vi "Average_data.vi"(7 "Data for averaging":dbl[][](array[numeric]), 8 "error in (no error)":errorcluster, 9 "Number to average":i32, 10 "New data":dbl[](array[numeric]), 11 "Gage digitizer actor in":refnum<class "Gage digitizer actor.lvclass">) -> (0 "error out":errorcluster, 2 "Aveage data":dbl[](array[numeric]), 3 "Gage digitizer actor out":refnum<class "Gage digitizer actor.lvclass">)   [LabVIEW 2015, in "Gage digitizer actor.lvclass"]
uses:
  Gage digitizer actor.lvclass
  <vilib>/Analysis/baseanly.llb/Mean (DBL).vi
  <vilib>/Analysis/NI_AALBase.lvlib
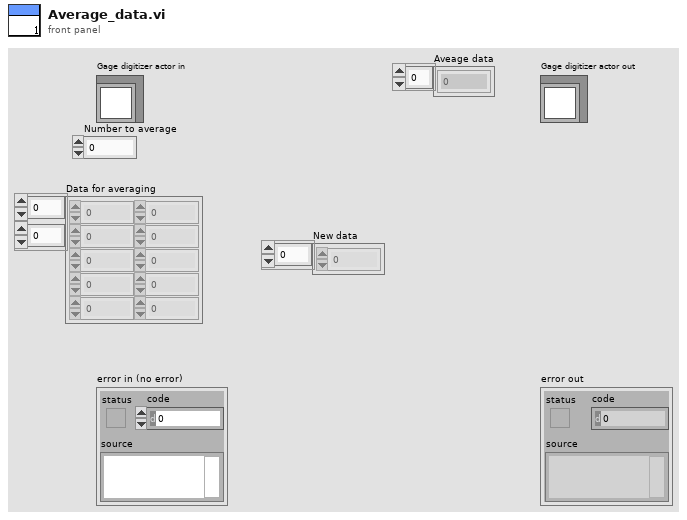
[diagram p1: front panel]
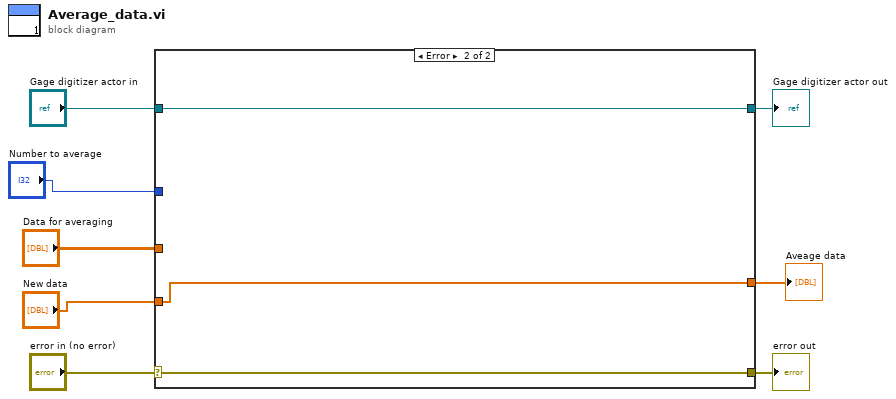
[diagram p0: block diagram]
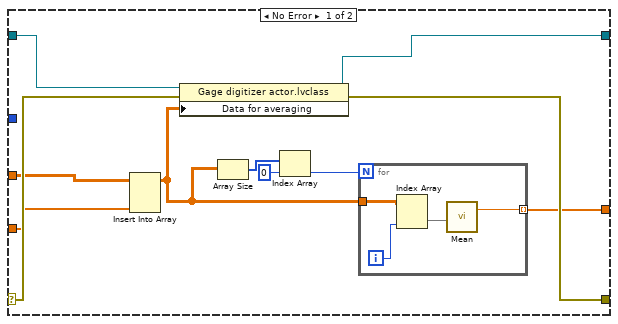
[diagram p2: hidden frame]
diagram:
  n1 = case shown="Error" "error in (no error)" {
    selector: "error in (no error)" -> [w17 w26]
    tunnel: [w16 w26] -> w7
    tunnel: [w18 w25] -> w5
    tunnel: "Gage digitizer actor in" -> [w19 w25]
    tunnel: "Data for averaging" -> [w15 _]
    tunnel: "Number to average" -> [_ _]
    tunnel: "New data" -> [w14 w24]
    tunnel: [w9 w24] -> w1
    frame No Error {
      n2 = Insert Into Array(array=w15, new element=w14) -> (w13:dbl[][])  [unwired: 2 in]
      n3 = property class="Gage digitizer actor.lvclass"(reference=w19, error in=w17, "Data for averaging"=w13) -> (reference out=w18:refnum<class "Gage digitizer actor.lvclass">, error out=w16:errorcluster)
      n4 = Array Size(array=w13) -> (size(s)=w12:i32[])
      n5 = Index Array(array=w12, index=0) -> (element=w10:i32)
      n6 = for {
        N: w10 -> [_]
        tunnel: w13 -> [w23]
        tunnel: [w20] -> w9 mode=indexing
        i -> [w22]
        n7 = Index Array(array=w23, index (col)=w22) -> (element=w21:dbl[])  [unwired: 1 in]
        n8 = call-poly <vilib>:"Mean.vi"("X"=w21) -> ("mean"=w20:dbl)  [unwired: 1 out]
      }
    }
    frame Error {
    }
  }
  "error out" <- w7
  "Gage digitizer actor out" <- w5
  "Aveage data" <- w1
